vi "Read configuration.vi"(8 "error in":errorcluster, 11 "ScaleAndLimitModule editor node in":refnum<class "ScaleAndLimitModule editor node.lvclass">) -> (0 "error out":errorcluster, 2 "configuration":refnum<class "NISE_CEF_serializable configuration.lvclass">, 3 "ScaleAndLimitModule editor node out":refnum<class "ScaleAndLimitModule editor node.lvclass">)   [LabVIEW 2017, in "ScaleAndLimitModule editor node.lvclass"]
uses:
  ScaleAndLimitModule editor node.lvclass
  <vilib>/NI/Configuration Framework/serializable configuration/NISE_CEF_serializable configuration.lvclass
  ScaleAndLimitModule editor node.lvclass/ScaleAndLimitModule editor node.ctl
  module/configuration/ScaleAndLimitModule configuration.lvclass
  C:/Program Files (x86)/National Instruments/LabVIEW 2017/vi.lib/NI/Configuration Framework/serializable configuration/NISE_CEF_serializable configuration.lvclass
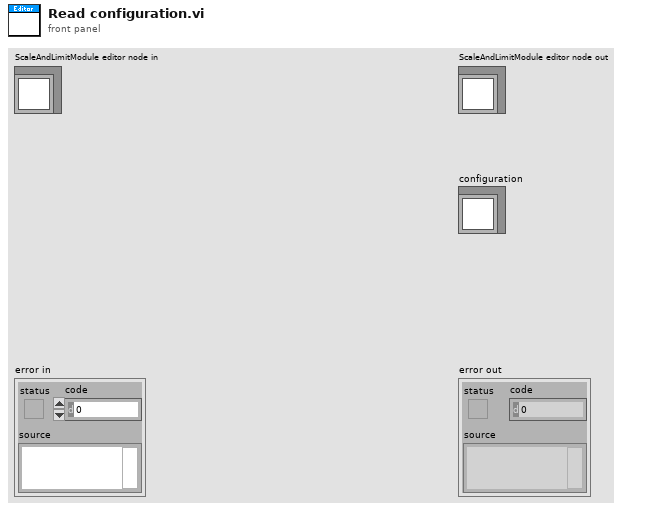
[diagram p1: front panel]
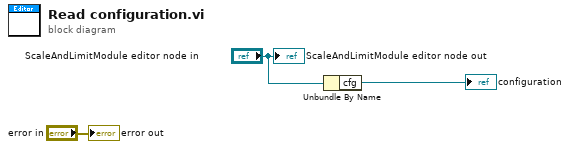
[diagram p0: block diagram]
diagram:
  n1 = Unbundle By Name("ScaleAndLimitModule editor node in") -> ("cfg"=→"configuration":refnum<class "ScaleAndLimitModule configuration.lvclass">)
  "error out" <- "error in"
  "ScaleAndLimitModule editor node out" <- "ScaleAndLimitModule editor node in"
